vi "WPI_RobotDriveMecanumDrive_Cartesian - Close loop 2252.vi"(0 "RobotDriveDevRef":T2={"DevStatus"={"status"=FALSE, "code"=0, "source"=""}, "Motors[]"=[], "Square Inputs"=FALSE, "Max Output"=1.0}, 1 "Gyro Angle":dbl, 2 "Encoder Front Left":dbl, 3 "Encoder Front Right":dbl, 5 "X (-1 to 1)":dbl, 7 "PID gains":T1 {"derivative time (Td, min)" format="%.3f"; "integral time (Ti, min)" format="%.3f"; "proportional gain (Kc)" format="%.3f"}, 9 "Y (-1 to 1)":dbl, 11 "error in (no error)":errorcluster, 12 "Rotation":dbl, 13 "Encoder Rear Left":dbl, 14 "Encoder Rear Right":dbl) -> (4 "RobotDriveDevRef":T2={"DevStatus"={"status"=FALSE, "code"=0, "source"=""}, "Motors[]"=[], "Square Inputs"=FALSE, "Max Output"=1.0}, 6 "Motor Values":dbl[](array[numeric]), 15 "error out":errorcluster)   [LabVIEW 2014]
doc: "Configures the motors for holonomic driving. Holonomic driving allows you to move the robot in any direction without first rotating or maneuvering the robot.\n\nThis VI requires the robot to have either four omni-directional wheels and four motors mounted at 45 degree angles in the four corners of a square frame or to have four mecanum wheels driven by four motors.\n\nThe control input is intended to be connected directly to the X, Y, and Z axes of a joystick. The Y axis is inverted for you.\n\nThis software is licensed. Open the labview\\readme\\WPI Robotics Library Open Source License.txt file for more information."
uses:
  <vilib>/Rock Robotics/WPI/RobotDrive/WPI_RobotDriveDevRef.ctl
  <vilib>/Rock Robotics/WPI/MotorControl/WPI_MotorControlDeviceRef.ctl
  <vilib>/Rock Robotics/WPI/MotorControl/WPI_MotorControlType.ctl
  <vilib>/Rock Robotics/SystemInterfaces/Typedef/FPGA_TypedefDigitalModule.ctl
  <vilib>/Rock Robotics/SystemInterfaces/DIO/FPGA_DIOPWMChannel.ctl
  <vilib>/Rock Robotics/WPI/PWM/WPI_PWMDeadband.ctl
  <vilib>/Rock Robotics/WPI/CAN/Jaguar/SubVIs/WPI_CANJaguar_ControlMode.ctl
  <vilib>/Rock Robotics/WPI/CAN/TalonSRX/WPI_CANTalonSRX_APIControlMode.ctl
  <vilib>/Rock Robotics/WPI/PWM/WPI_PWMTransform_ConPane.ctl
  <vilib>/Rock Robotics/SystemInterfaces/NetworkCommunication/NetComm_UsageReport_ResourceType.ctl
  <vilib>/Rock Robotics/WPI/RobotDrive/WPI_RobotDriveMotorSelectorEnum.ctl
  <vilib>/Rock Robotics/WPI/RobotDrive/WPI_RobotDriveSafetyCheck.vi
panel:
  out "Y'":dbl(graph)
  in  "Offset Factor":dbl
  in  "output range":cluster{"output high":dbl, "output low":dbl}={"output high"=1.0, "output low"=-1.0} {"output low" format="%.2f"; "output high" format="%.2f"}
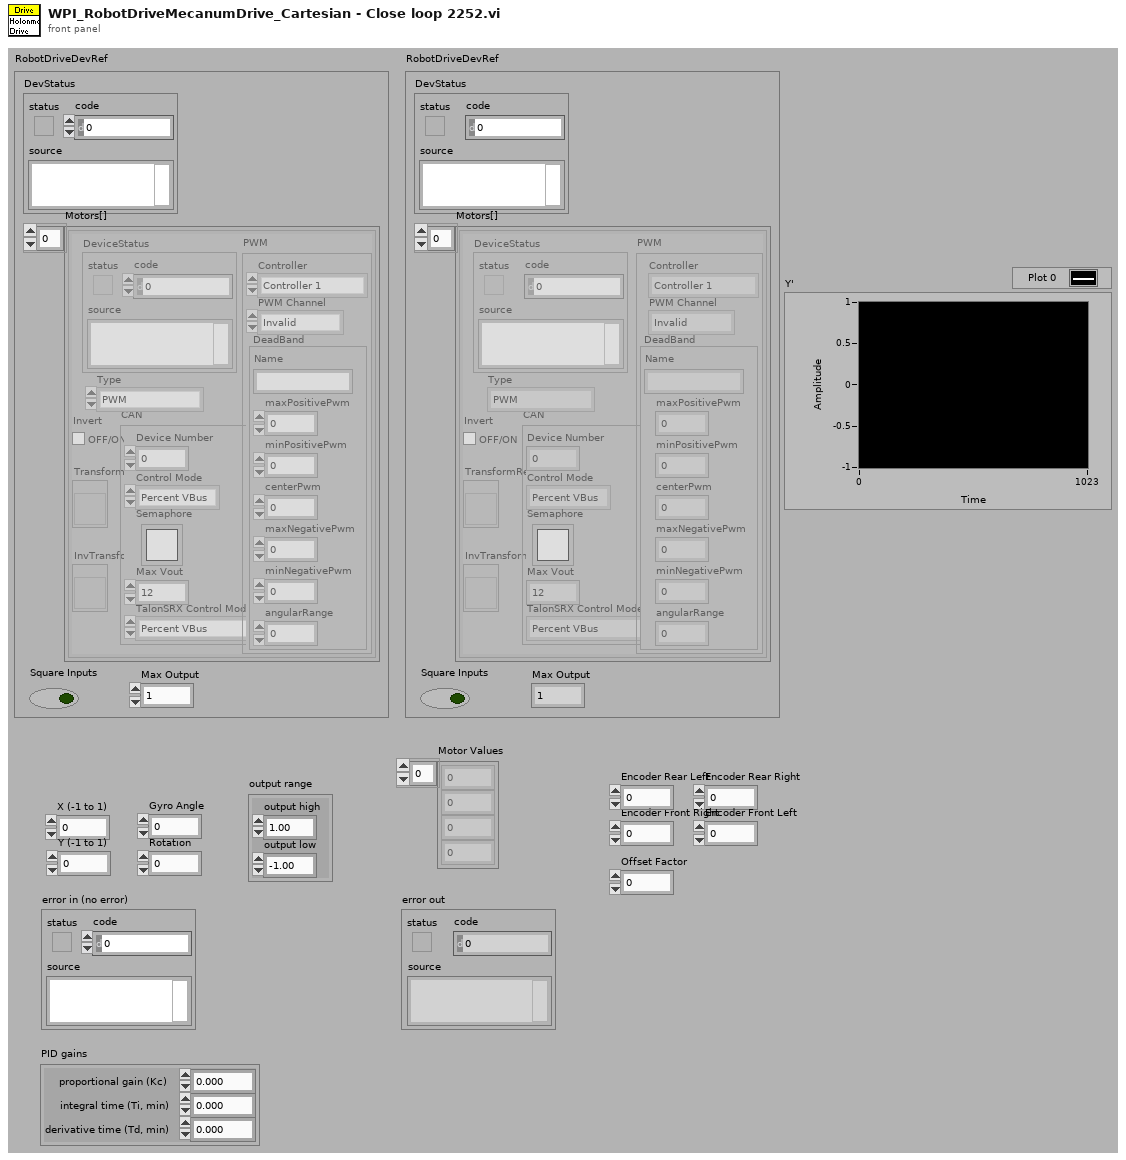
[diagram p1: front panel]
types:
  T1 = cluster{"proportional gain (Kc)":dbl, "integral time (Ti, min)":dbl, "derivative time (Td, min)":dbl}
  T2 = typedef "WPI_RobotDriveDevRef.ctl" = cluster{"DevStatus":errorcluster, "Motors[]":T3[], "Square Inputs":bool, "Max Output":dbl}
  T3 = typedef "WPI_MotorControlDeviceRef.ctl" = cluster{"DeviceStatus":errorcluster, "Type":T4, "PWM":cluster{"Controller":T5, "PWM Channel":T6, "DeadBand":T7}, "CAN":cluster{"Device Number":u8, "Control Mode":T8, "Semaphore":T9, "Max Vout":dbl, "TalonSRX Control Mode":T10}, "Invert":bool, "TransformRef":T11, "InvTransformRef":T11}
  T4 = typedef "WPI_MotorControlType.ctl" = enum16{"PWM", "CAN", "CANTalonSRX"}
  T5 = typedef "FPGA_TypedefDigitalModule.ctl" = enum16{"Controller 1"}
  T6 = typedef "FPGA_DIOPWMChannel.ctl" = enum8{"PWM 0", "PWM 1", "PWM 2", "PWM 3", "PWM 4", "PWM 5", "PWM 6", "PWM 7", "PWM 8", "PWM 9", "PWM MXP 0", "PWM MXP 1", "PWM MXP 2", "PWM MXP 3", "PWM MXP 4", "PWM MXP 5", "PWM MXP 6", "PWM MXP 7", "PWM MXP 8", "PWM MXP 9", "Invalid"}
  T7 = typedef "WPI_PWMDeadband.ctl" = cluster{"Name":string, "maxPositivePwm":i32, "minPositivePwm":i32, "centerPwm":i32, "maxNegativePwm":i32, "minNegativePwm":i32, "angularRange":u16}
  T8 = typedef "WPI_CANJaguar_ControlMode.ctl" = enum8{"Percent VBus", "Current", "Speed", "Position", "Voltage"}
  T9 = typedef "Semaphore RefNum" = refnum<k1>
  T10 = typedef "WPI_CANTalonSRX_APIControlMode.ctl" = enum8{"Percent VBus", "Speed", "Position", "Slave", "Unchanged / Invalid"}
  T11 = typedef "WPI_PWMTransform_ConPane.ctl" = refnum<vi>
  T12 = typedef "NetComm_UsageReport_ResourceType.ctl" = enum8{"Controller", "Module", "Language", "CANPlugin", "Accelerometer", "ADXL345", "AnalogChannel", "AnalogTrigger", "AnalogTriggerOutput", "CANJaguar", "Compressor", "Counter", "Dashboard", "DigitalInput", "DigitalOutput", "DriverStationCIO", "DriverStationEIO", "DriverStationLCD", "Encoder", "GearTooth", "Gyro", "I2C", "Framework", "Jaguar", "Joystick", "Kinect", "KinectStick", "PIDController", "Preferences", "PWM", "Relay", "RobotDrive", "SerialPort", "Servo", "Solenoid", "SPI", "Task", "Ultrasonic", "Victor", "Button", "Command", "AxisCamera", "PCVideoServer", "SmartDashboard", "Talon", "HiTechnicColorSensor", "HiTechnicAccel", "HiTechnicCompass", "SRF08", "AnalogOutput", "Victor SP", "Talon SRX", "CAN Talon SRX"}
  T13 = typedef "WPI_RobotDriveMotorSelectorEnum.ctl" = enum16{"Rear Left Motor", "Rear Right Motor", "Front Left Motor", "Front Right Motor"}
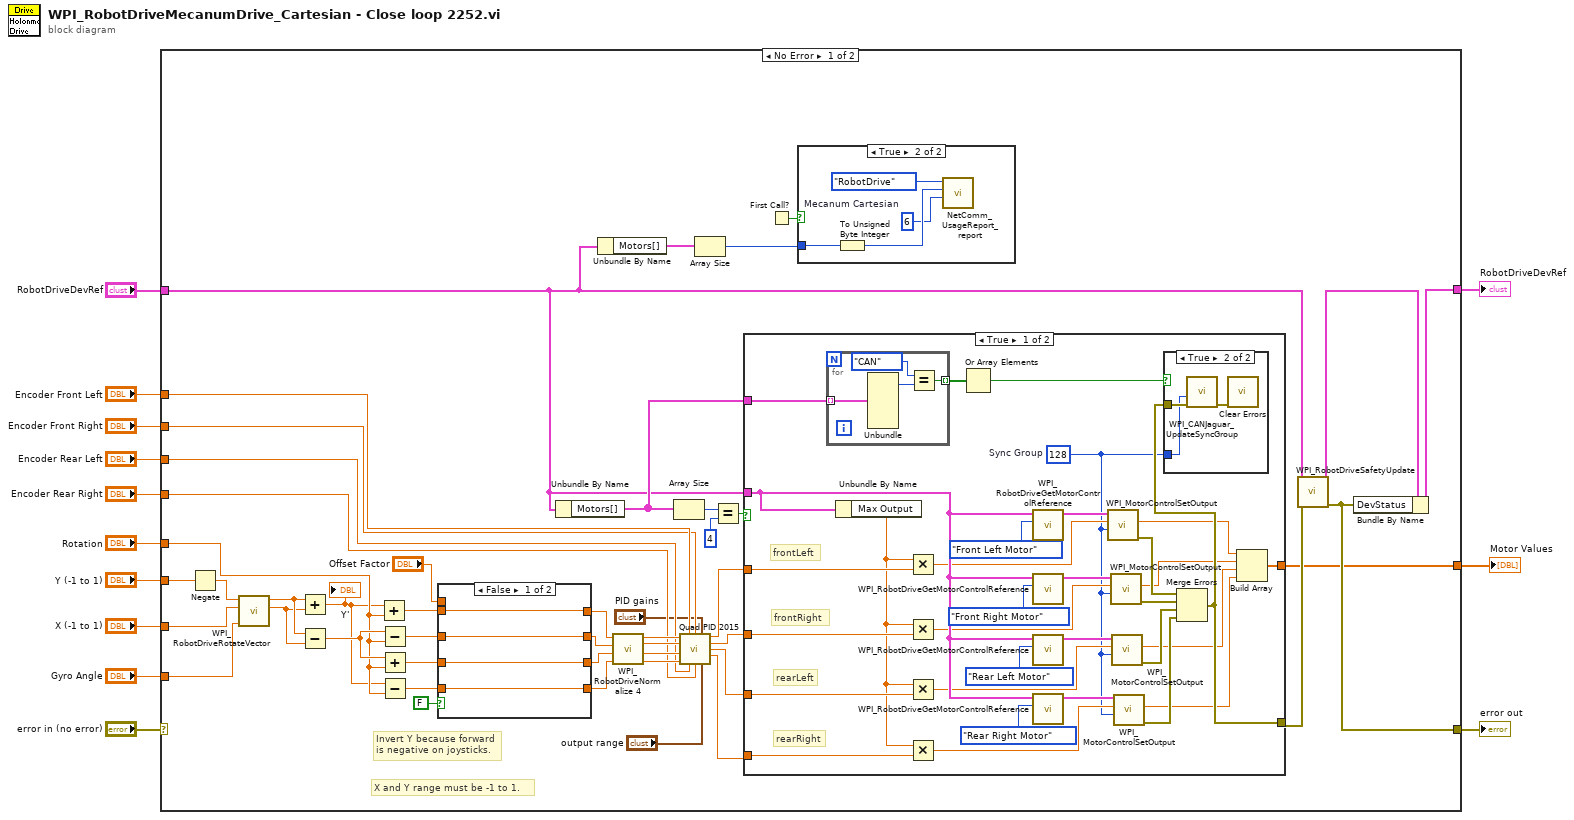
[diagram p0: block diagram]
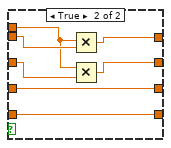
[diagram p2: hidden frame]
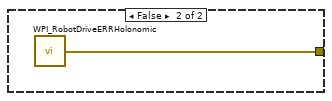
[diagram p5: hidden frame]
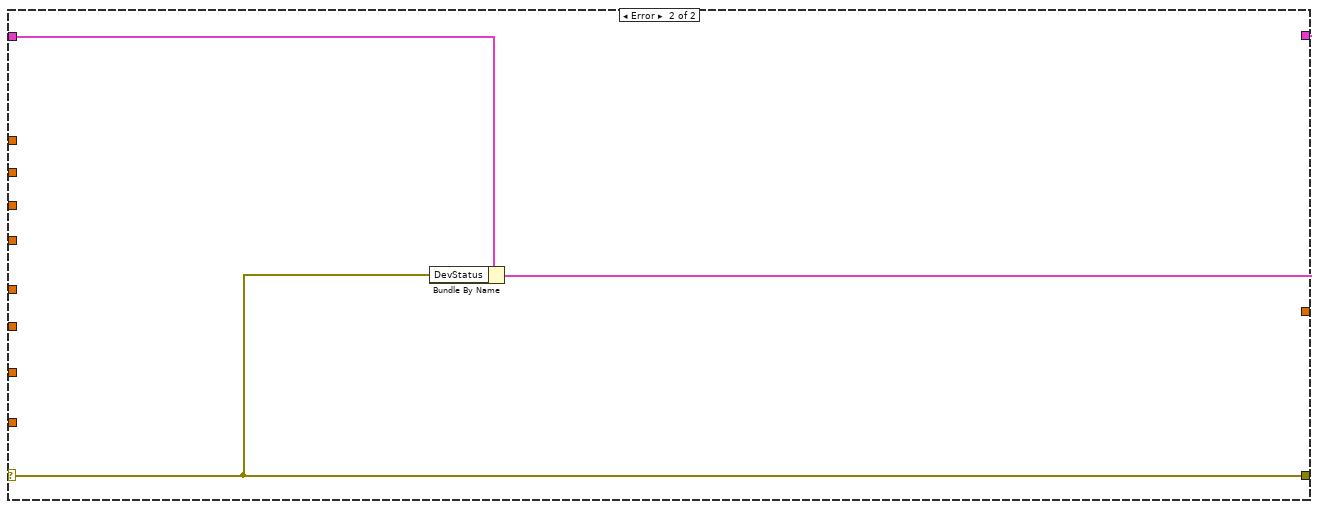
[diagram p6: hidden frame]
diagram:
  n1 = case shown="No Error" "error in (no error)" {
    selector: "error in (no error)" -> [_ w115]
    tunnel: "Y (-1 to 1)" -> [w51 _]
    tunnel: "X (-1 to 1)" -> [w52 _]
    tunnel: "RobotDriveDevRef" -> [w41 w117]
    tunnel: [w56 w116] -> w9
    tunnel: [w46 w115] -> w8
    tunnel: "Rotation" -> [w35 _]
    tunnel: "Gyro Angle" -> [w50 _]
    tunnel: [w40 _] -> w5
    tunnel: "Encoder Front Left" -> [w34 _]
    tunnel: "Encoder Front Right" -> [w33 _]
    tunnel: "Encoder Rear Left" -> [w32 _]
    tunnel: "Encoder Rear Right" -> [w31 _]
    frame No Error {
      # "X and Y range must be -1 to 1."
      # "Invert Y because forward is negative on joysticks."
      n2 = Negate(x=w51) -> (-x=w49:dbl)
      n3 = call <vilib>:"WPI_RobotDriveRotateVector.vi"("Angle"=w50, "X"=w52, "Y"=w49) -> ("X'"=w54:dbl, "Y'"=w55:dbl)  [unwired: 7 out]
      n4 = Add(x=w55, y=w54) -> (x+y=w14:dbl)
      "Y'" <- w14
      n5 = Subtract(x=w55, y=w54) -> (x-y=w53:dbl)
      n6 = Add(x=w14, y=w35) -> (x+y=w15:dbl)
      n7 = Subtract(x=w53, y=w35) -> (x-y=w23:dbl)
      n8 = Add(x=w53, y=w35) -> (x+y=w21:dbl)
      n9 = Subtract(x=w14, y=w35) -> (x-y=w18:dbl)
      n10 = case shown="False" FALSE {
        tunnel: w15 -> [w63 w65]
        tunnel: [w63 w67] -> w24
        tunnel: w23 -> [w62 w66]
        tunnel: [w62 w68] -> w22
        tunnel: w21 -> [w61 w70]
        tunnel: [w61 w70] -> w20
        tunnel: [w60 w69] -> w19
        tunnel: w18 -> [w60 w69]
        tunnel: "Offset Factor" -> [_ w64]
        frame False {
        }
        frame True {
          n11 = Multiply(x=w64, y=w65) -> (x*y=w67:dbl)
          n12 = Multiply(x=w64, y=w66) -> (x*y=w68:dbl)
        }
      }
      n13 = Unbundle By Name(w41) -> ("Motors[]"=w45:T3[])
      n14 = Unbundle By Name(w41) -> ("Motors[]"=w43:T3[])
      n15 = call <vilib>:"WPI_RobotDriveNormalize 4.vi"("D"=w19, "C"=w20, "B"=w22, "A"=w24) -> ("D'"=w36:dbl, "C'"=w37:dbl, "B'"=w38:dbl, "A'"=w39:dbl)
      n16 = Array Size(array=w45) -> (size(s)=w59:i32)
      n17 = call "Quad PID 2015.vi"("Target Velocity (rev/sec) 1"=w39, "Measured Velocity (rev/sec) 1"=w34, "Measured Velocity (rev/sec) 2"=w33, "PID gains"="PID gains", "Target Velocity (rev/sec) 2"=w38, "Target Velocity (rev/sec) 3"=w37, "Target Velocity (rev/sec) 4"=w36, "Measured Velocity (rev/sec) 3"=w32, "Measured Velocity (rev/sec) 4"=w31, "output range"="output range") -> ("Output Value (-1 to +1) 1"=w28:dbl, "Output Value (-1 to +1) 2"=w27:dbl, "Output Value (-1 to +1) 3"=w26:dbl, "Output Value (-1 to +1) 4"=w25:dbl)  [unwired: 2 in]
      n18 = Array Size(array=w43) -> (size(s)=w42:i32)
      n19 = Equal?(x=w59, y=4) -> (x = y?=w57:bool)
      n20 = case shown="True" w57 {
        tunnel: w28 -> [w106 _]
        tunnel: w27 -> [w105 _]
        tunnel: w41 -> [w94 _]
        tunnel: [w81 w114] -> w48
        tunnel: w26 -> [w100 _]
        tunnel: w25 -> [w99 _]
        tunnel: w45 -> [w82 _]
        tunnel: [w78 _] -> w40
        frame True {
          w80 = u8 128  # Sync Group
          # "rearLeft"
          # "frontRight"
          # "rearRight"
          # "frontLeft"
          n21 = for {
            tunnel: w82 -> [w110] mode=indexing
            tunnel: [w107] -> w83 mode=indexing
            n22 = Unbundle(w110) -> ("Type"=w109:T4)  [unwired: 6 out]
            n23 = Equal?(x=enum16{"PWM", "CAN"}."CAN" ("Type"), y=w109) -> (x = y?=w107:bool)
          }
          n24 = Unbundle By Name(w94) -> ("Max Output"=w89:dbl)
          n25 = Multiply(x=w89, y=w106) -> (x*y=w93:dbl)
          n26 = Multiply(x=w89, y=w105) -> (x*y=w92:dbl)
          n27 = Multiply(x=w89, y=w100) -> (x*y=w91:dbl)
          n28 = Multiply(x=w89, y=w99) -> (x*y=w90:dbl)
          n29 = Or Array Elements(Boolean array=w83) -> (logical OR=w84:bool)
          n30 = call <vilib>:"WPI_RobotDriveGetMotorControlReference.vi"("MotorIndex"=WPI_RobotDriveMotorSelectorEnum."Front Left Motor", "RobotDriveDevRef"=w94) -> ("MotorControlDeviceRef"=w104:T3)  [unwired: 9 out]
          n31 = call <vilib>:"WPI_RobotDriveGetMotorControlReference.vi"("MotorIndex"=WPI_RobotDriveMotorSelectorEnum."Front Right Motor", "RobotDriveDevRef"=w94) -> ("MotorControlDeviceRef"=w102:T3)  [unwired: 9 out]
          n32 = call <vilib>:"WPI_RobotDriveGetMotorControlReference.vi"("MotorIndex"=WPI_RobotDriveMotorSelectorEnum."Rear Left Motor", "RobotDriveDevRef"=w94) -> ("MotorControlDeviceRef"=w103:T3)  [unwired: 9 out]
          n33 = call <vilib>:"WPI_RobotDriveGetMotorControlReference.vi"("MotorIndex"=WPI_RobotDriveMotorSelectorEnum."Rear Right Motor", "RobotDriveDevRef"=w94) -> ("MotorControlDeviceRef"=w101:T3)  [unwired: 9 out]
          n34 = call <vilib>:"WPI_MotorControlSetOutput.vi"("Sync Group / Parameter Slot"=w80, "Output"=w93, "MotorControlDevRef"=w104) -> ("error out"=w85:errorcluster, "Motor Output"=w79:dbl)  [unwired: 2 in, 5 out]
          n35 = call <vilib>:"WPI_MotorControlSetOutput.vi"("Sync Group / Parameter Slot"=w80, "Output"=w92, "MotorControlDevRef"=w102) -> ("error out"=w86:errorcluster, "Motor Output"=w77:dbl)  [unwired: 2 in, 5 out]
          n36 = call <vilib>:"WPI_MotorControlSetOutput.vi"("Sync Group / Parameter Slot"=w80, "Output"=w91, "MotorControlDevRef"=w103) -> ("error out"=w87:errorcluster, "Motor Output"=w76:dbl)  [unwired: 2 in, 5 out]
          n37 = call <vilib>:"WPI_MotorControlSetOutput.vi"("Sync Group / Parameter Slot"=w80, "Output"=w90, "MotorControlDevRef"=w101) -> ("error out"=w88:errorcluster, "Motor Output"=w75:dbl)  [unwired: 2 in, 5 out]
          n38 = Merge Errors(w85, w86, w87, w88) -> (w81:errorcluster)
          n39 = case shown="True" w84 {
            tunnel: w81 -> [_ w112]
            tunnel: w80 -> [_ w111]
            frame False {
            }
            frame True {
              n40 = call <vilib>:"WPI_CANJaguar_UpdateSyncGroup.vi"("error in (no error)"=w112, "Sync Group"=w111) -> ("error out"=w113:errorcluster)  [unwired: 9 out]
              n41 = call <vilib>:"Clear Errors.vi"("error in (no error)"=w113) -> ()  [unwired: 1 in, 6 out]
            }
          }
          n42 = Build Array(w79, w77, w76, w75) -> (w78:dbl[])
        }
        frame False {
          n43 = call <vilib>:"WPI_RobotDriveERRHolonomic.vi"() -> ("error out"=w114:errorcluster)
        }
      }
      n44 = First Call?() -> (First Call?: T/F=w44:bool)
      n45 = case shown="True" w44 {
        tunnel: w42 -> [_ w73]
        frame False {
        }
        frame True {
          w71 = u8 6  # Mecanum Cartesian
          n46 = To Unsigned Byte Integer(number=w73) -> (unsigned 8bit integer=w72:u8)
          n47 = call <vilib>:"NetComm_UsageReport_report.vi"("Context"=w71, "Instance Number"=w72, "Resource Type"=NetComm_UsageReport_ResourceType."RobotDrive") -> ()  [unwired: 9 in]
        }
      }
      n48 = call <vilib>:"WPI_RobotDriveSafetyUpdate.vi"("error in (no error)"=w48, "RobotDriveDevRef"=w41) -> ("error out"=w46:errorcluster, "RobotDriveDevRef"=w47:T2)  [unwired: 8 out]
      n49 = Bundle By Name(cluster=w47, "DevStatus"=w46) -> (w56:T2)
    }
    frame Error {
      n50 = Bundle By Name(cluster=w117, "DevStatus"=w115) -> (w116:T2)
    }
  }
  "error out" <- w8
  "RobotDriveDevRef" <- w9
  "Motor Values" <- w5
